vi "ROI_Image_Create tangent line to circle.vi"(8 "error in (no error)":errorcluster, 9 "Orient rel to center":T2, 10 "Circles Data":T4, 11 "Intersection Point":cluster{"X":i32, "Y":i32}) -> (0 "error out":errorcluster, 1 "Line End Points":cluster{"X":dbl, "Y":dbl}[](array[cluster]), 2 "Tangent Line":T3 {"Point 2"."Y" format="%.2f"; "Point 2"."X" format="%.2f"; "Point 1"."Y" format="%.2f"; "Point 1"."X" format="%.2f"}, 4 "ROI":T1 {"Contours"."Type" items=["No Selection", "Point", "Line", "Rectangle", "Oval", "Polygon", "Freehand Region", "Annulus", "Unused2", "Unused3", "Broken Line", "Freehand Line", "Rotated Rectangle"]})   [LabVIEW 2014]
uses:
  custom controls/enum - StartPt Relative to Circle Center.ctl
  FileIO/TypeDef - File Actions.ctl
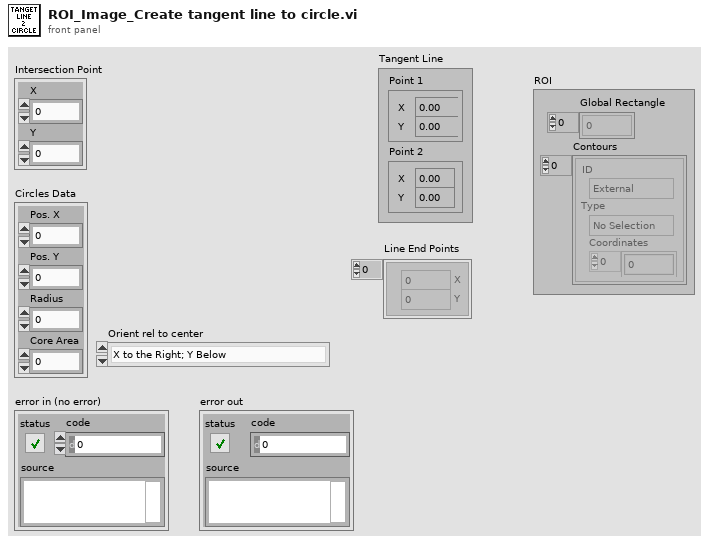
[diagram p1: front panel]
types:
  T1 = typedef "ROI Descriptor" = cluster{"Global Rectangle":i32[], "Contours":cluster{"ID":enum32{"External", "Internal"}, "Type":u32, "Coordinates":i32[]}[]}
  T2 = typedef "enum - StartPt Relative to Circle Center.ctl" = enum16{"X to the Right; Y Below", "X to the Right; Y Above", "X to the Left; Y Below", "X to the Left: Y Above"}
  T3 = cluster{"Point 1":cluster{"X":sgl, "Y":sgl}, "Point 2":cluster{"X":sgl, "Y":sgl}}
  T4 = cluster{"Pos. X":i32, "Pos. Y":i32, "Radius":i32, "Core Area":i32}
  T5 = typedef "TypeDef - File Actions.ctl" = enum16{"Read", "Write", "Get Current"}
  T6 = cluster{"ID":enum32{"External", "Internal"}, "Type":u32, "Coordinates":i32[]}
  T7 = typedef "TypeDef - System Configuration.ctl" = cluster{"Results FilePath":path, "Analysis Parameters":cluster{"Area":cluster{"Lower Value":dbl, "Upper Value":dbl}, "Circle Filter Radius":cluster{"Lower Value":sgl, "Upper Value":sgl}, "Edge Detection Threshold":u16}, "ROI Parameters":cluster{"ROI size (in Radius)":cluster{"Width":dbl, "Height":dbl}}}
  T8 = cluster{"ID":enum32{"External", "Internal"}, "Type":u32, "Coordinates":i32[]}[]
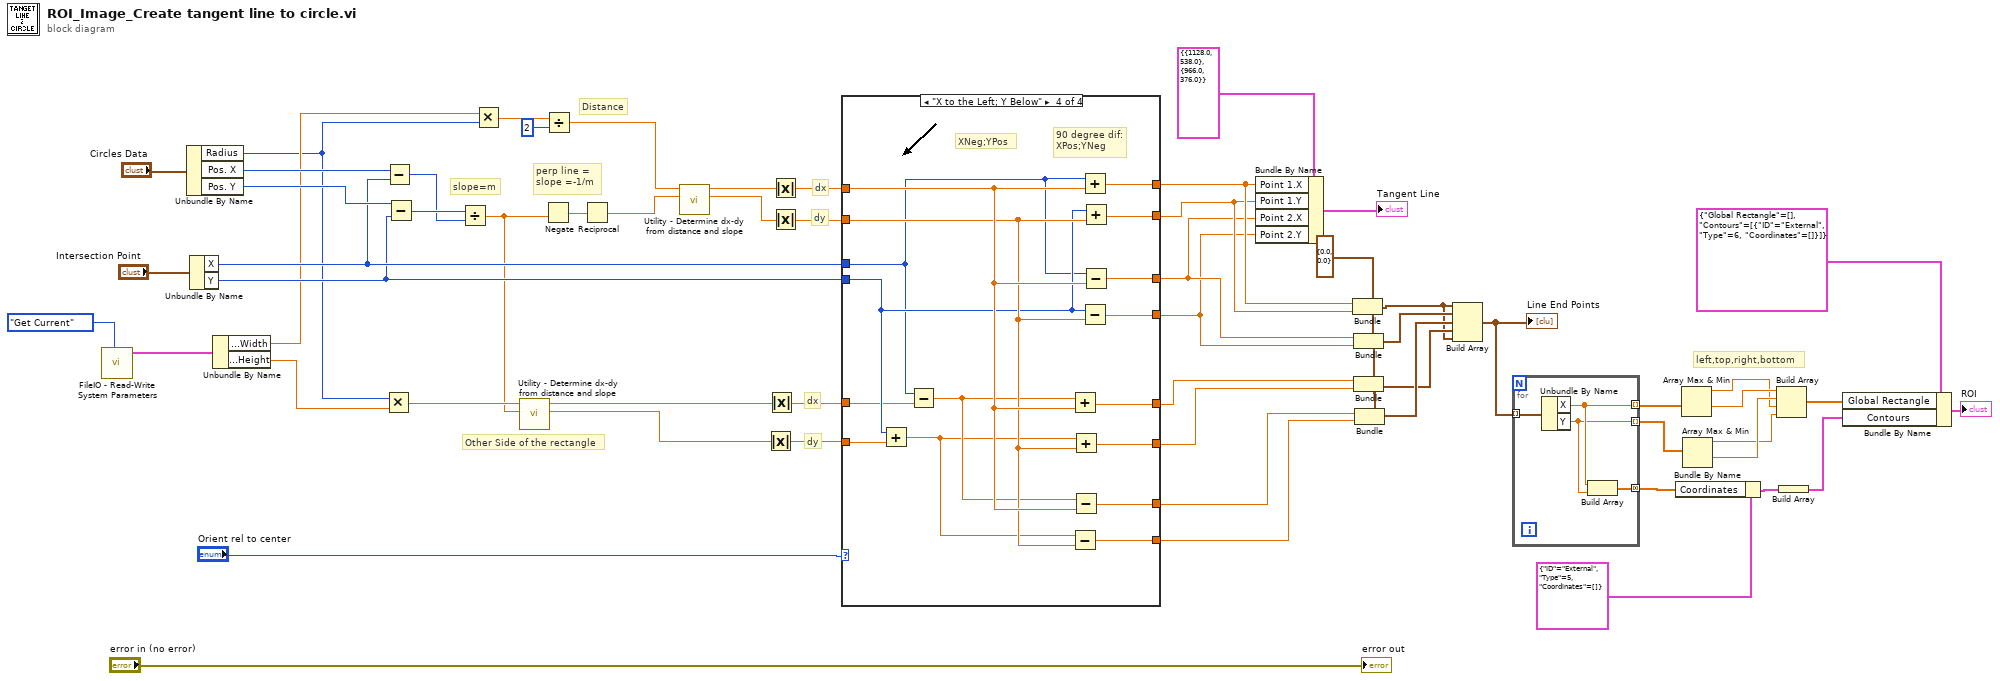
[diagram p0: block diagram]
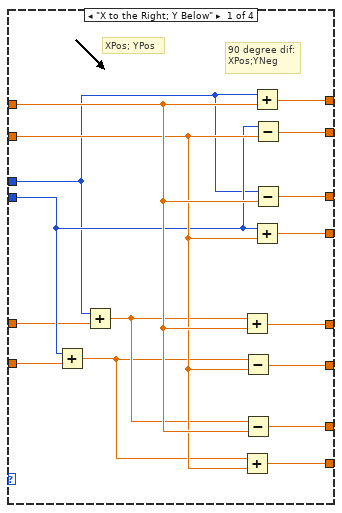
[diagram p2: hidden frame]
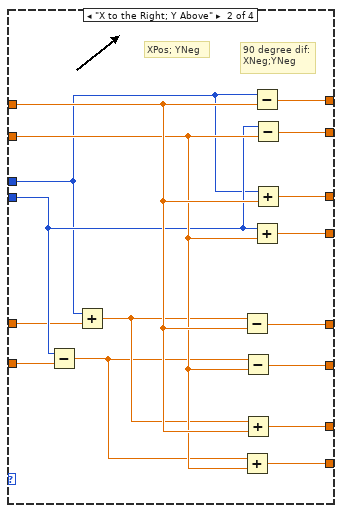
[diagram p3: hidden frame]
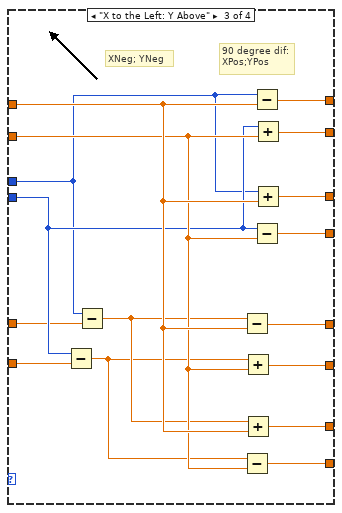
[diagram p4: hidden frame]
diagram:
  w22 = cluster{"X":dbl, "Y":dbl} {"X"=0.0, "Y"=0.0} ("Point Coordinates")
  # "left,top,right,bottom"
  # "Distance"
  # "dx"
  # "Other Side of the rectangle"
  # "dy"
  # "dy"
  # "dx"
  # "perp line =  \nslope =-1/m"
  # "slope=m"
  n1 = call "FileIO - Read-Write System Parameters.vi"("Action"=TypeDef_-_File_Actions."Get Current") -> ("System Parameters out"=w5:T7)  [unwired: 9 in, 1 out]
  n2 = Unbundle By Name("Circles Data") -> ("Radius"=w1:i32, "Pos. X"=w56:i32, "Pos. Y"=w55:i32)
  n3 = Unbundle By Name("Intersection Point") -> ("X"=w47:i32, "Y"=w32:i32)
  n4 = Unbundle By Name(w5) -> ("ROI Parameters.ROI size (in Radius).Width"=w2:dbl, "ROI Parameters.ROI size (in Radius).Height"=w4:dbl)
  n5 = Multiply(x=w1, y=w4) -> (x*y=w28:dbl)
  n6 = Subtract(x=w56, y=w47) -> (x-y=w53:i32)
  n7 = Subtract(x=w55, y=w32) -> (x-y=w54:i32)
  n8 = Divide(x=w54, y=w53) -> (x/y=w27:dbl)
  n9 = Multiply(x=w2, y=w1) -> (x*y=w3:dbl)
  n10 = call "Utility - Determine dx-dy from distance and slope.vi"("Slope (dy/dx)"=w27, "Distance= r"=w28) -> ("dy"=w25:dbl, "dx"=w26:dbl)  [unwired: 8 in]
  n11 = Negate(x=w27) -> (-x=w52:dbl)
  n12 = Divide(x=w3, y=2) -> (x/y=w46:dbl)
  n13 = Reciprocal(x=w52) -> (1/x=w50:dbl)
  n14 = call "Utility - Determine dx-dy from distance and slope.vi"("Slope (dy/dx)"=w50, "Distance= r"=w46) -> ("dy"=w45:dbl, "dx"=w29:dbl)  [unwired: 8 in]
  n15 = Absolute Value(x=w25) -> (abs(x)=w24:dbl)
  n16 = Absolute Value(x=w26) -> (abs(x)=w31:dbl)
  n17 = Absolute Value(x=w29) -> (abs(x)=w23:dbl)
  n18 = Absolute Value(x=w45) -> (abs(x)=w30:dbl)
  n19 = case shown="\"X to the Left; Y Below\"" "Orient rel to center" {
    tunnel: w47 -> [w63 w79 w95 w111]
    tunnel: w32 -> [w64 w80 w96 w112]
    tunnel: w23 -> [w75 w91 w107 w123]
    tunnel: w30 -> [w74 w90 w106 w122]
    tunnel: [w73 w89 w105 w121] -> w44
    tunnel: [w72 w88 w104 w120] -> w43
    tunnel: [w71 w87 w103 w119] -> w42
    tunnel: [w70 w86 w102 w118] -> w41
    tunnel: [w69 w85 w101 w117] -> w39
    tunnel: [w68 w84 w100 w116] -> w38
    tunnel: [w67 w83 w99 w115] -> w37
    tunnel: [w66 w82 w98 w114] -> w36
    tunnel: w24 -> [w65 w81 w97 w113]
    tunnel: w31 -> [w62 w78 w94 w110]
    frame "X to the Right; Y Below" {
      # "90 degree dif:\nXPos;YNeg"
      # "XPos; YPos"
      n20 = Add(x=w64, y=w65) -> (x+y=w60:dbl)
      n21 = Add(x=w63, y=w62) -> (x+y=w61:dbl)
      n22 = Add(x=w61, y=w75) -> (x+y=w69:dbl)
      n23 = Add(x=w60, y=w74) -> (x+y=w66:dbl)
      n24 = Subtract(x=w60, y=w74) -> (x-y=w68:dbl)
      n25 = Subtract(x=w61, y=w75) -> (x-y=w67:dbl)
      n26 = Add(x=w63, y=w75) -> (x+y=w73:dbl)
      n27 = Add(x=w64, y=w74) -> (x+y=w70:dbl)
      n28 = Subtract(x=w64, y=w74) -> (x-y=w72:dbl)
      n29 = Subtract(x=w63, y=w75) -> (x-y=w71:dbl)
    }
    frame "X to the Right; Y Above" {
      # "90 degree dif:\nXNeg;YNeg"
      # "XPos; YNeg"
      n30 = Subtract(x=w80, y=w81) -> (x-y=w76:dbl)
      n31 = Add(x=w79, y=w78) -> (x+y=w77:dbl)
      n32 = Subtract(x=w77, y=w91) -> (x-y=w85:dbl)
      n33 = Add(x=w76, y=w90) -> (x+y=w82:dbl)
      n34 = Subtract(x=w76, y=w90) -> (x-y=w84:dbl)
      n35 = Add(x=w77, y=w91) -> (x+y=w83:dbl)
      n36 = Subtract(x=w79, y=w91) -> (x-y=w89:dbl)
      n37 = Add(x=w80, y=w90) -> (x+y=w86:dbl)
      n38 = Subtract(x=w80, y=w90) -> (x-y=w88:dbl)
      n39 = Add(x=w79, y=w91) -> (x+y=w87:dbl)
    }
    frame "X to the Left: Y Above" {
      # "90 degree dif:\nXPos;YPos"
      # "XNeg; YNeg"
      n40 = Subtract(x=w96, y=w97) -> (x-y=w92:dbl)
      n41 = Subtract(x=w95, y=w94) -> (x-y=w93:dbl)
      n42 = Subtract(x=w93, y=w107) -> (x-y=w101:dbl)
      n43 = Subtract(x=w92, y=w106) -> (x-y=w98:dbl)
      n44 = Add(x=w92, y=w106) -> (x+y=w100:dbl)
      n45 = Add(x=w93, y=w107) -> (x+y=w99:dbl)
      n46 = Subtract(x=w95, y=w107) -> (x-y=w105:dbl)
      n47 = Subtract(x=w96, y=w106) -> (x-y=w102:dbl)
      n48 = Add(x=w96, y=w106) -> (x+y=w104:dbl)
      n49 = Add(x=w95, y=w107) -> (x+y=w103:dbl)
    }
    frame "X to the Left; Y Below" {
      # "90 degree dif:\nXPos;YNeg"
      # "XNeg;YPos"
      n50 = Add(x=w112, y=w113) -> (x+y=w108:dbl)
      n51 = Subtract(x=w111, y=w110) -> (x-y=w109:dbl)
      n52 = Add(x=w109, y=w123) -> (x+y=w117:dbl)
      n53 = Subtract(x=w108, y=w122) -> (x-y=w114:dbl)
      n54 = Add(x=w108, y=w122) -> (x+y=w116:dbl)
      n55 = Subtract(x=w109, y=w123) -> (x-y=w115:dbl)
      n56 = Add(x=w111, y=w123) -> (x+y=w121:dbl)
      n57 = Subtract(x=w112, y=w122) -> (x-y=w118:dbl)
      n58 = Add(x=w112, y=w122) -> (x+y=w120:dbl)
      n59 = Subtract(x=w111, y=w123) -> (x-y=w119:dbl)
    }
  }
  n60 = Bundle By Name(cluster=T3 {"Point 1"={"X"=1128.0, "Y"=538.0}, "Point 2"={"X"=966.0, "Y"=376.0}} ("Tangent Line"), "Point 1.X"=w44, "Point 1.Y"=w43, "Point 2.X"=w42, "Point 2.Y"=w41) -> (→"Tangent Line":T3)
  n61 = Bundle(cluster=w22, "X"=w44, "Y"=w43) -> (w8:cluster{"X":dbl, "Y":dbl})
  n62 = Bundle(cluster=w22, "X"=w42, "Y"=w41) -> (w40:cluster{"X":dbl, "Y":dbl})
  n63 = Bundle(cluster=w22, "X"=w39, "Y"=w38) -> (w34:cluster{"X":dbl, "Y":dbl})
  n64 = Bundle(cluster=w22, "X"=w37, "Y"=w36) -> (w35:cluster{"X":dbl, "Y":dbl})
  n65 = Build Array(w8, w40, w35, w34, w8) -> (w7:cluster{"X":dbl, "Y":dbl}[])
  "Line End Points" <- w7
  n66 = for {
    tunnel: w7 -> [w127] mode=indexing
    tunnel: [w126] -> w21 mode=indexing
    tunnel: [w125] -> w20 mode=indexing
    tunnel: [w124] -> w12 mode=concatenating
    n67 = Unbundle By Name(w127) -> ("X"=w126:dbl, "Y"=w125:dbl)
    n68 = Build Array(w126, w125) -> (w124:dbl[])
  }
  n69 = Bundle By Name(cluster=T6 {"ID"=enum."External", "Type"=5, "Coordinates"=[]}, "Coordinates"=w12) -> (w11:T6)
  n70 = Array Max & Min(array=w21) -> (max value=w17:dbl, min value=w19:dbl)  [unwired: 2 out]
  n71 = Array Max & Min(array=w20) -> (max value=w16:dbl, min value=w18:dbl)  [unwired: 2 out]
  n72 = Build Array(w19, w18, w17, w16) -> (w14:dbl[])
  n73 = Build Array(w11) -> (w10:T8)
  n74 = Bundle By Name(cluster=T1 {"Global Rectangle"=[], "Contours"=[{"ID"=enum."External", "Type"=6, "Coordinates"=[]}]} ("ROI Descriptor"), "Global Rectangle"=w14, "Contours"=w10) -> (→"ROI":T1)
  "error out" <- "error in (no error)"
